vi "IgnoredFailCountDetails_RC.vi"(8 "error in (no error)":errorcluster, 10 "IgnoredCountDetails":cluster{"ReelCount":u64, "TotalCount":u64}, 11 "Rack Controller in":refnum<class "Rack Controller.lvclass">) -> (0 "error out":errorcluster, 3 "Rack Controller out":refnum<class "Rack Controller.lvclass">)   [LabVIEW 2019, in "Rack Controller.lvclass"]
uses:
  Rack Controller.lvclass
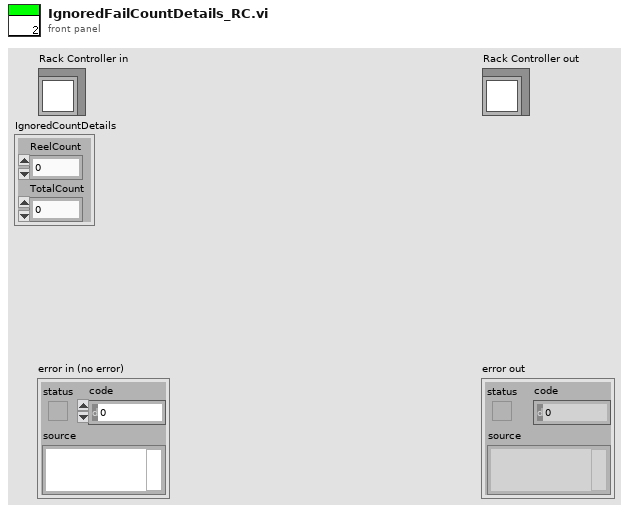
[diagram p1: front panel]
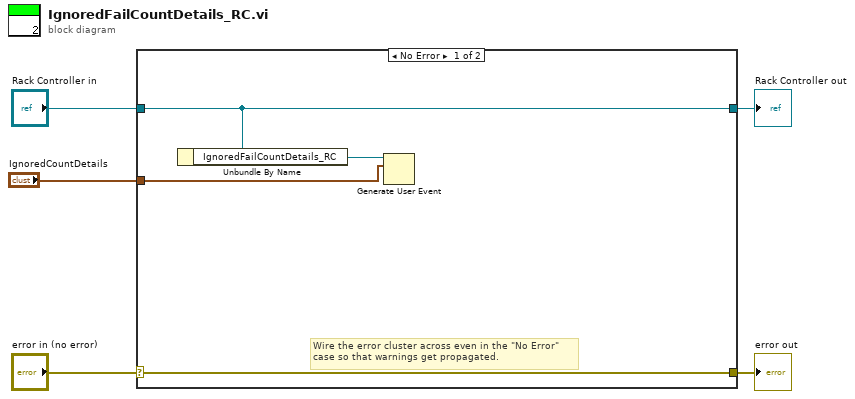
[diagram p0: block diagram]
diagram:
  n1 = case shown="No Error" "error in (no error)" {
    selector: "error in (no error)" -> [w9 w11]
    tunnel: [w9 w11] -> w4
    tunnel: [w8 w10] -> w2
    tunnel: "Rack Controller in" -> [w8 w10]
    tunnel: "IgnoredCountDetails" -> [w6 _]
    frame No Error {
      # "Wire the error cluster across even in the \"No Error\"\ncase so that warnings get propagated."
      n2 = Unbundle By Name(w8) -> ("IgnoredFailCountDetails_RC"=w7:refnum<user-event>)
      n3 = Generate User Event(user event=w7, event data cluster=w6) -> ()  [unwired: 2 in, 2 out]
    }
    frame Error {
    }
  }
  "error out" <- w4
  "Rack Controller out" <- w2
